vi "MeasureIV.vi"(5 "Junction Name":string, 6 "UiDefinition":T1, 7 ".NET Refnum":refnum<k24>, 8 "new file path (Not A Path if cancelled)":path, 9 "appended path":path, 11 ".NET Refnum in":refnum<k24>) -> (0 "error out":errorcluster)   [LabVIEW 2020]
uses:
  C:/Users/User/Desktop/Automation/CurrentVersion/LabviewDXFViewer/bin/Release/LabviewDXFViewer.exe
  LabviewDXFViewer/bin/Release/LabviewDXFViewer.exe
  UIReferences.ctl
  <vilib>/Utility/file.llb/Write Delimited Spreadsheet (string).vi
  <vilib>/Utility/file.llb/Write Delimited Spreadsheet (DBL).vi
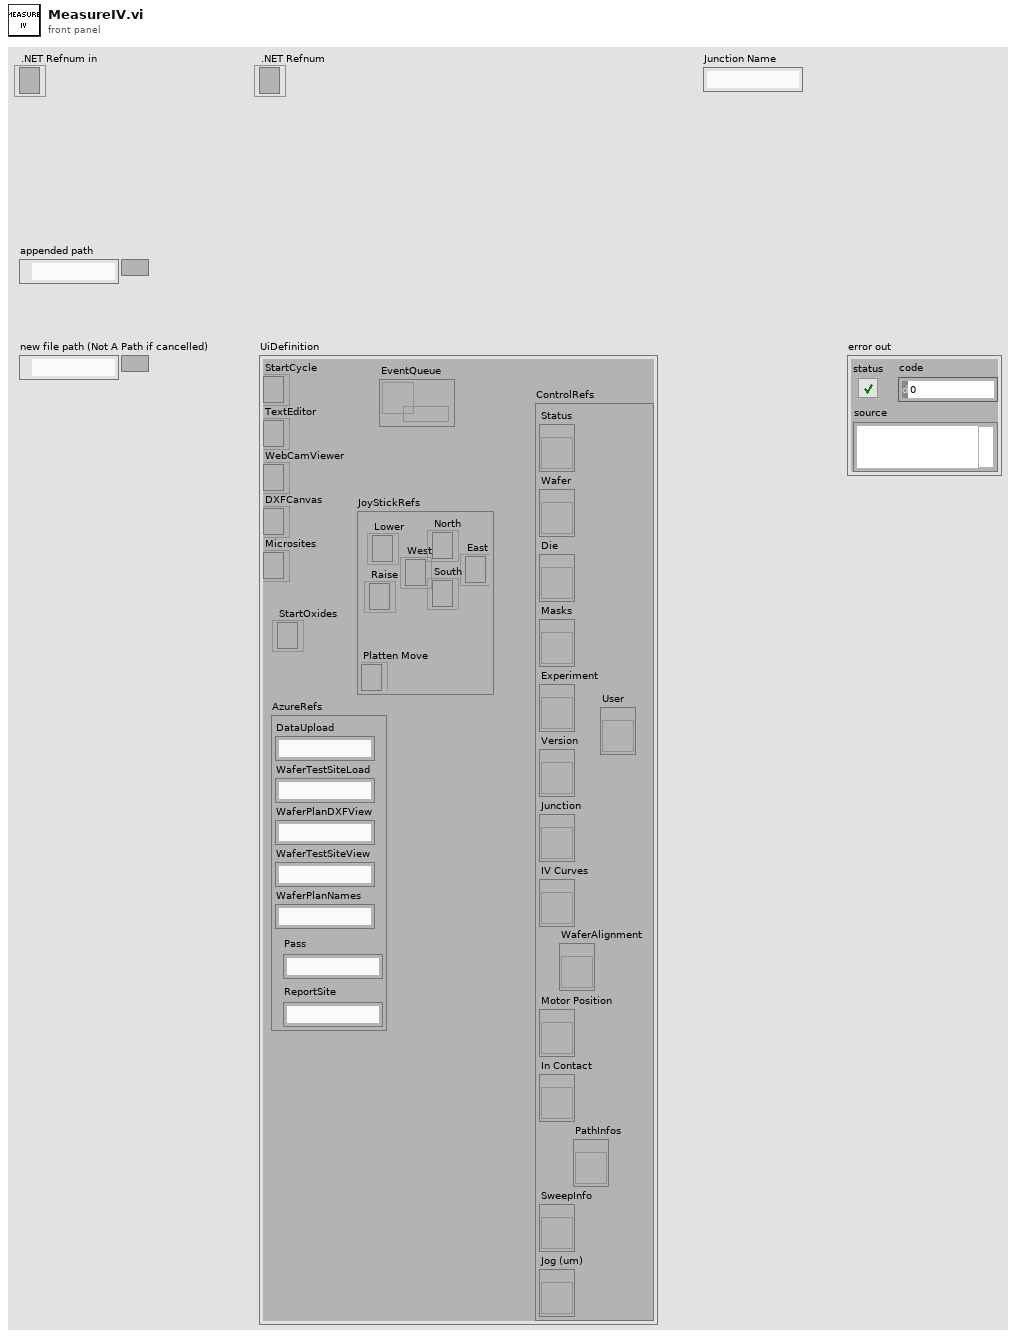
[diagram p1: front panel]
types:
  T1 = typedef "UIReferences.ctl" = cluster{"StartCycle":refnum<k24>, "TextEditor":refnum<k24>, "WebCamViewer":refnum<k24>, "DXFCanvas":refnum<k24>, "Microsites":refnum<k24>, "JoyStickRefs":cluster{"North":refnum<k24>, "Lower":refnum<k24>, "Raise":refnum<k24>, "Platten Move":refnum<k24>, "West":refnum<k24>, "East":refnum<k24>, "South":refnum<k24>}, "AzureRefs":cluster{"DataUpload":string, "WaferTestSiteLoad":string, "WaferPlanDXFView":string, "WaferTestSiteView":string, "WaferPlanNames":string, "Pass":string, "ReportSite":string}, "ControlRefs":cluster{"Status":refnum<vi>, "Wafer":refnum<vi>, "Die":refnum<vi>, "Masks":refnum<vi>, "Experiment":refnum<vi>, "Version":refnum<vi>, "Junction":refnum<vi>, "IV Curves":refnum<vi>, "Motor Position":refnum<vi>, "In Contact":refnum<vi>, "SweepInfo":refnum<vi>, "Jog (um)":refnum<vi>, "PathInfos":refnum<vi>, "User":refnum<vi>, "WaferAlignment":refnum<vi>}, "EventQueue":refnum<queue>, "StartOxides":refnum<k24>}
  T2 = typedef "CapacitanceInfos.ctl" = cluster{"Conductance":dbl, "CapacitanceIV":dbl, "Intercept":dbl, "CapacitanceSW":dbl, "Sum":dbl, "CapacitanceInfos":T3[], "CapacitancePhase":dbl, "dC/dV":dbl, "Function":string, "OtherInfo":dbl[][]}
  T3 = typedef "CapacitanceRecord.ctl" = cluster{"Freq":dbl, "Vpp":dbl, "PhaseS":dbl, "Irms":dbl, "PhaseC":dbl, "Theta":dbl, "VDrive":dbl, "Capacitance":dbl, "Other":dbl}
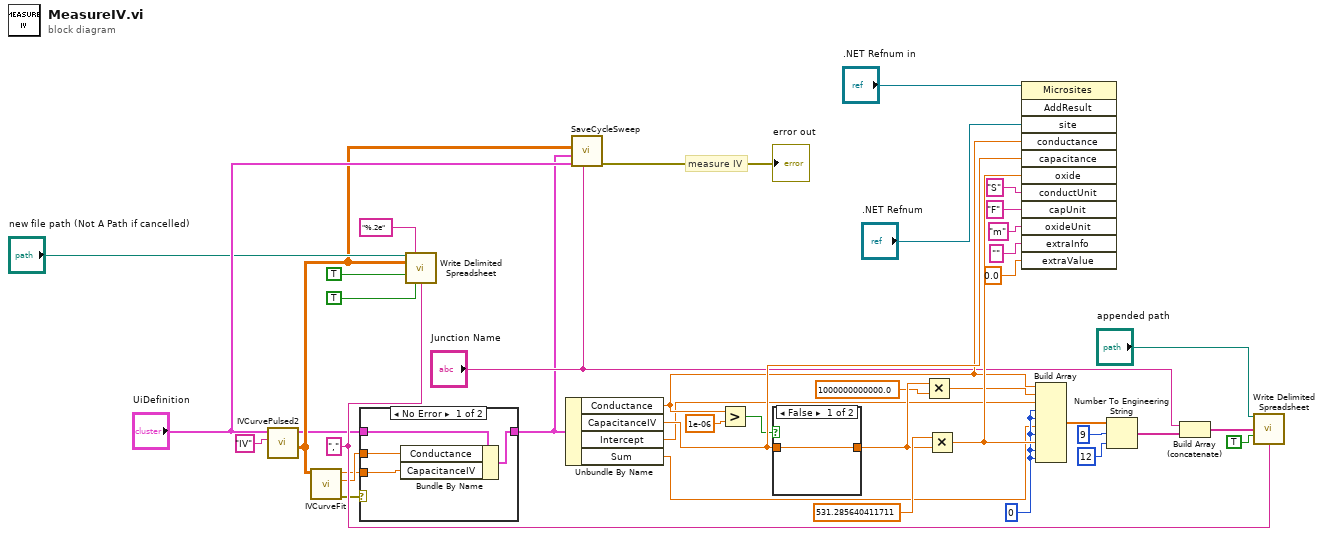
[diagram p0: block diagram]
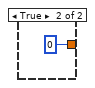
[diagram p3: hidden frame]
diagram:
  w10 = "," ("delimiter (\\t)")
  w36 = 0
  # "measure IV"
  n1 = call "IVCurvePulsed2.vi"("Program"="IV", "UiDefinition"="UiDefinition") -> ("appended array"=w6:dbl[][], "InfoCluster"=w4:T2)  [unwired: 8 in]
  n2 = call "IVCurveFit.vi"("IVData"=w6) -> ("error out"=w5:errorcluster, "Conductance"=w3:dbl, "Capacitance"=w2:dbl)  [unwired: 7 in, 1 out]
  n3 = case shown="No Error" w5 {
    tunnel: w4 -> [w45 w46]
    tunnel: w3 -> [w44 _]
    tunnel: w2 -> [w43 _]
    tunnel: [w42 w46] -> w1
    frame No Error {
      n4 = Bundle By Name(cluster=w45, "Conductance"=w44, "CapacitanceIV"=w43) -> (w42:T2)
    }
    frame Error {
    }
  }
  n5 = call-poly <vilib>:"Write Delimited Spreadsheet.vi"("file path (dialog if empty)"="new file path (Not A Path if cancelled)", "format (%.3f)"="%.2e", "2D data"=w6, "append to file? (new file:F)"=TRUE, "transpose? (no:F)"=TRUE, "delimiter (\\t)"=w10) -> ()  [unwired: 8 in, 2 out]
  n6 = Unbundle By Name(w1) -> ("Conductance"=w37:dbl, "CapacitanceIV"=w38:dbl, "Intercept"=w20:dbl, "Sum"=w21:dbl)
  n7 = call "SaveCycleSweep.vi"("JunctionName"="Junction Name", "UiDefinition 2"="UiDefinition", "InfoCluster"=w1, "appended array"=w6) -> ("error out"=→"error out":errorcluster)  [unwired: 7 in]
  n8 = Greater?(x=w37, y=1e-06) -> (0:w24:bool)
  n9 = case shown="False" w24 {
    tunnel: [w47 0] -> w39
    tunnel: w38 -> [w47 _]
    frame False {
    }
    frame True {
    }
  }
  n10 = Multiply(x=w39, y=1000000000000.0) -> (x*y=w22:dbl)
  n11 = Multiply(x=531.285640411711, y=w39) -> (x*y=w41:dbl)
  n12 = invoke class="Microsites" method="AddResult"(reference=".NET Refnum in", "site"=".NET Refnum", "conductance"=w37, "capacitance"=w38, "oxide"=w41, "conductUnit"="S", "capUnit"="F", "oxideUnit"="m" ("interceptUnit"), "extraInfo"="", "extraValue"=0.0) -> ()  [unwired: 2 in, 12 out]
  n13 = Build Array(w37, w22, w20, w36, w36, w21, w36, w41, w36, w36) -> (w19:dbl[])
  n14 = Number To Engineering String(2:i16 12 ("precision (6)"), 3:i16 9 ("width (-)"), 4:w19) -> (0:w12:string[])  [unwired: 1 in]
  n15 = Build Array (concatenate)("Junction Name", w12) -> (w14:string[])
  n16 = call-poly <vilib>:"Write Delimited Spreadsheet.vi"("file path (dialog if empty)"="appended path", "1D data"=w14, "append to file? (new file:F)"=TRUE, "delimiter (\\t)"=w10) -> ()  [unwired: 10 in, 2 out]
